vi "DC Basic Measure.vi"(4 "Channel 2":bool, 5 "Voltmeter 2 Address":string="8", 6 "Channel 1":bool=TRUE, 7 "Voltmeter 1 Address":string="7", 9 "Period (s)":string="1", 10 "Amplitude (A)":string="1e-8") -> (0 "STD 2":dbl=0.00015789614384998, 1 "Resistance 2":dbl=0.023133111600000002, 2 "STD 1":dbl=1.1063759259570055e-05, 3 "Resistance 1":dbl=0.04676234421500001)   [LabVIEW 2020]
uses:
  <vilib>/Instr/_visa.llb/GPIB Status Boolean Array.ctl
panel:
  out "Buffer 2 Data":dbl[][](array[numeric])=[[0.0, 1.69853343e-06], [0.05, 2.29085744e-06], [0.101, 2.2689427e-06], [0.152, 2.25641999e-06], [0.203, 2.27896086e-06], [0.254, 2.27332565e-06], [0.305, 2.24828023e-06], [0.356, 2.26142908e-06], [0.407, 2.27708246e-06], [0.458, 2.26268135e-06], [0.509, 2.28146541e-06], [0.56, 2.27520405e-06], [0.611, 2.25266318e-06], [0.662, 2.27207338e-06], [0.713, 2.26268135e-06], [0.764, 2.26455975e-06], [0.815, 2.27457792e-06], [0.866, 2.25892453e-06], [0.917, 2.28021313e-06], [0.968, 2.27144724e-06], [1.019, 2.2495325e-06], [1.07, 2.24201888e-06], [1.121, 2.2476541e-06], [1.172, 2.23763593e-06], [1.223, 2.25203705e-06], [1.274, 2.22260869e-06], [1.325, 2.25892453e-06], [1.376, 2.2689427e-06], [1.427, 2.23262685e-06], [1.478, 1.17257976e-06], [1.529, -2.35755925e-06], [1.58, -2.36006378e-06], [1.631, -2.37696934e-06], [1.681, -2.35192407e-06], [1.731, -2.35630699e-06], [1.781, -2.34628888e-06], [1.832, -2.35881152e-06], [1.882, -2.33188785e-06], [1.932, -2.33814917e-06], [1.982, -2.34941954e-06], [2.032, -2.3368969e-06], [2.083, -2.3782216e-06], [2.133, -2.36131604e-06], [2.183, -2.33752304e-06], [2.233, -2.36256831e-06], [2.283, -2.38135226e-06], [2.333, -2.36757736e-06], [2.384, -2.36068991e-06], [2.434, -2.37133415e-06], [2.484, -2.3782216e-06], [2.534, -2.3763432e-06], [2.584, -2.37696934e-06], [2.635, -2.37133415e-06], [2.685, -2.40264074e-06], [2.735, -2.37321255e-06], [2.785, -2.3801e-06], [2.835, -2.37947386e-06], [2.885, -2.38636131e-06], [2.935, -2.36882962e-06], [2.985, -1.36075749e-06], [3.035, -5.33931926e-08], [3.085, -3.6487539e-08]]
  out "Buffer 2 Plot":cluster{dbl[], dbl[]}(graph)={[0.0, 0.05, 0.101, 0.152, 0.203, 0.254, 0.305, 0.356, 0.407, 0.458, 0.509, 0.56, 0.611, 0.662, 0.713, 0.764, 0.815, 0.866, 0.917, 0.968, 1.019, 1.07, 1.121, 1.172, 1.223, 1.274, 1.325, 1.376, 1.427, 1.478, 1.529, 1.58, 1.631, 1.681, 1.731, 1.781, 1.832, 1.882, 1.932, 1.982, 2.032, 2.083, 2.133, 2.183, 2.233, 2.283, 2.333, 2.384, 2.434, 2.484, 2.534, 2.584, 2.635, 2.685, 2.735, 2.785, 2.835, 2.885, 2.935, 2.985, 3.035, 3.085], [1.69853343e-06, 2.29085744e-06, 2.2689427e-06, 2.25641999e-06, 2.27896086e-06, 2.27332565e-06, 2.24828023e-06, 2.26142908e-06, 2.27708246e-06, 2.26268135e-06, 2.28146541e-06, 2.27520405e-06, 2.25266318e-06, 2.27207338e-06, 2.26268135e-06, 2.26455975e-06, 2.27457792e-06, 2.25892453e-06, 2.28021313e-06, 2.27144724e-06, 2.2495325e-06, 2.24201888e-06, 2.2476541e-06, 2.23763593e-06, 2.25203705e-06, 2.22260869e-06, 2.25892453e-06, 2.2689427e-06, 2.23262685e-06, 1.17257976e-06, -2.35755925e-06, -2.36006378e-06, -2.37696934e-06, -2.35192407e-06, -2.35630699e-06, -2.34628888e-06, -2.35881152e-06, -2.33188785e-06, -2.33814917e-06, -2.34941954e-06, -2.3368969e-06, -2.3782216e-06, -2.36131604e-06, -2.33752304e-06, -2.36256831e-06, -2.38135226e-06, -2.36757736e-06, -2.36068991e-06, -2.37133415e-06, -2.3782216e-06, -2.3763432e-06, -2.37696934e-06, -2.37133415e-06, -2.40264074e-06, -2.37321255e-06, -2.3801e-06, -2.37947386e-06, -2.38636131e-06, -2.36882962e-06, -1.36075749e-06, -5.33931926e-08, -3.6487539e-08]}
  out "Voltage 2":dbl[](array[numeric])=[2.31331116e-06, 1.5789614384998e-08]
  out "Python error 2":errorcluster
  out "T2":dbl[](array[numeric])=[0.0, 0.05, 0.101, 0.152, 0.203, 0.254, 0.305, 0.356, 0.407, 0.458, 0.509, 0.56, 0.611, 0.662, 0.713, 0.764, 0.815, 0.866, 0.917, 0.968, 1.019, 1.07, 1.121, 1.172, 1.223, 1.274, 1.325, 1.376, 1.427, 1.478, 1.529, 1.58, 1.631, 1.681, 1.731, 1.781, 1.832, 1.882, 1.932, 1.982, 2.032, 2.083, 2.133, 2.183, 2.233, 2.283, 2.333, 2.384, 2.434, 2.484, 2.534, 2.584, 2.635, 2.685, 2.735, 2.785, 2.835, 2.885, 2.935, 2.985, 3.035, 3.085]
  out "V2":dbl[](array[numeric])=[1.69853343e-06, 2.29085744e-06, 2.2689427e-06, 2.25641999e-06, 2.27896086e-06, 2.27332565e-06, 2.24828023e-06, 2.26142908e-06, 2.27708246e-06, 2.26268135e-06, 2.28146541e-06, 2.27520405e-06, 2.25266318e-06, 2.27207338e-06, 2.26268135e-06, 2.26455975e-06, 2.27457792e-06, 2.25892453e-06, 2.28021313e-06, 2.27144724e-06, 2.2495325e-06, 2.24201888e-06, 2.2476541e-06, 2.23763593e-06, 2.25203705e-06, 2.22260869e-06, 2.25892453e-06, 2.2689427e-06, 2.23262685e-06, 1.17257976e-06, -2.35755925e-06, -2.36006378e-06, -2.37696934e-06, -2.35192407e-06, -2.35630699e-06, -2.34628888e-06, -2.35881152e-06, -2.33188785e-06, -2.33814917e-06, -2.34941954e-06, -2.3368969e-06, -2.3782216e-06, -2.36131604e-06, -2.33752304e-06, -2.36256831e-06, -2.38135226e-06, -2.36757736e-06, -2.36068991e-06, -2.37133415e-06, -2.3782216e-06, -2.3763432e-06, -2.37696934e-06, -2.37133415e-06, -2.40264074e-06, -2.37321255e-06, -2.3801e-06, -2.37947386e-06, -2.38636131e-06, -2.36882962e-06, -1.36075749e-06, -5.33931926e-08, -3.6487539e-08]
  out "Write Status 2":T1=[FALSE, FALSE, FALSE, FALSE, FALSE, FALSE, FALSE, FALSE, TRUE, FALSE, FALSE, FALSE, FALSE, FALSE, FALSE, FALSE]
  out "error out 2":errorcluster
  out "Read Status 2":T1=[FALSE, FALSE, FALSE, FALSE, FALSE, FALSE, FALSE, FALSE, TRUE, FALSE, FALSE, FALSE, FALSE, TRUE, FALSE, FALSE]
  out "Buffer 1 Data":dbl[][](array[numeric])=[[0.0, 9.9e+37], [0.014, 9.9e+37], [0.026, 9.9e+37], [0.04, 9.9e+37], [0.052, 9.9e+37], [0.067, 9.9e+37], [0.079, 9.9e+37], [0.093, 9.9e+37], [0.105, 9.9e+37], [0.12, 9.9e+37], [0.132, 9.9e+37], [0.146, 9.9e+37], [0.158, 9.9e+37], [0.172, 9.9e+37], [0.184, 9.9e+37], [0.199, 9.9e+37], [0.211, 9.9e+37], [0.225, 9.9e+37], [0.237, 9.9e+37], [0.251, 9.9e+37], [0.263, 9.9e+37], [0.277, 9.9e+37], [0.289, 9.9e+37], [0.304, 9.9e+37], [0.316, 9.9e+37], [0.33, 9.9e+37], [0.342, 9.9e+37], [0.356, 9.9e+37], [0.368, 9.9e+37], [0.383, 9.9e+37], [0.395, 9.9e+37], [0.409, 9.9e+37], [0.422, 9.9e+37], [0.437, 9.9e+37], [0.449, 9.9e+37], [0.463, 9.9e+37], [0.475, 9.9e+37], [0.49, 9.9e+37], [0.502, 9.9e+37], [0.516, 9.9e+37], [0.528, 9.9e+37], [0.542, 9.9e+37], [0.554, 9.9e+37], [0.568, 9.9e+37], [0.58, 9.9e+37], [0.595, 9.9e+37], [0.607, 9.9e+37], [0.621, 9.9e+37], [0.633, 9.9e+37], [0.647, 9.9e+37], [0.659, 9.9e+37], [0.674, 9.9e+37], [0.686, 9.9e+37], [0.7, 9.9e+37], [0.712, 9.9e+37], [0.726, 9.9e+37], [0.738, 9.9e+37], [0.753, 9.9e+37], [0.765, 9.9e+37], [0.779, 9.9e+37], [0.791, 9.9e+37], [0.805, 9.9e+37]]
  out "Buffer 1 Plot":cluster{dbl[], dbl[]}(graph)={[0.0, 0.014, 0.026, 0.04, 0.052, 0.067, 0.079, 0.093, 0.105, 0.12, 0.132, 0.146, 0.158, 0.172, 0.184, 0.199, 0.211, 0.225, 0.237, 0.251, 0.263, 0.277, 0.289, 0.304, 0.316, 0.33, 0.342, 0.356, 0.368, 0.383, 0.395, 0.409, 0.422, 0.437, 0.449, 0.463, 0.475, 0.49, 0.502, 0.516, 0.528, 0.542, 0.554, 0.568, 0.58, 0.595, 0.607, 0.621, 0.633, 0.647, 0.659, 0.674, 0.686, 0.7, 0.712, 0.726, 0.738, 0.753, 0.765, 0.779, 0.791, 0.805], [9.9e+37, 9.9e+37, 9.9e+37, 9.9e+37, 9.9e+37, 9.9e+37, 9.9e+37, 9.9e+37, 9.9e+37, 9.9e+37, 9.9e+37, 9.9e+37, 9.9e+37, 9.9e+37, 9.9e+37, 9.9e+37, 9.9e+37, 9.9e+37, 9.9e+37, 9.9e+37, 9.9e+37, 9.9e+37, 9.9e+37, 9.9e+37, 9.9e+37, 9.9e+37, 9.9e+37, 9.9e+37, 9.9e+37, 9.9e+37, 9.9e+37, 9.9e+37, 9.9e+37, 9.9e+37, 9.9e+37, 9.9e+37, 9.9e+37, 9.9e+37, 9.9e+37, 9.9e+37, 9.9e+37, 9.9e+37, 9.9e+37, 9.9e+37, 9.9e+37, 9.9e+37, 9.9e+37, 9.9e+37, 9.9e+37, 9.9e+37, 9.9e+37, 9.9e+37, 9.9e+37, 9.9e+37, 9.9e+37, 9.9e+37, 9.9e+37, 9.9e+37, 9.9e+37, 9.9e+37, 9.9e+37, 9.9e+37]}
  in  "Python Support File":path=path "C:/Users/QDUser/Desktop/LabVIEW Programs/PPMS Interface/lib/PPMS External Control Support.py"
  out "Voltage 1":dbl[](array[numeric])=[0.0, 0.014, 0.026, 0.04, 0.052, 0.067, 0.079, 0.093, 0.105, 0.12, 0.132, 0.146, 0.158, 0.172, 0.184, 0.199, 0.211, 0.225, 0.237, 0.251, 0.263, 0.277, 0.289, 0.304, 0.316, 0.33, 0.342, 0.356, 0.368, 0.383, 0.395, 0.409, 0.422, 0.437, 0.449, 0.463, 0.475, 0.49, 0.502, 0.516, 0.528, 0.542, 0.554, 0.568, 0.58, 0.595, 0.607, 0.621, 0.633, 0.647, 0.659, 0.674, 0.686, 0.7, 0.712, 0.726, 0.738, 0.753, 0.765, 0.779, 0.791, 0.805]
  out "Python error":errorcluster={"status"=TRUE, "code"=1671, "source"="Python Node in DC Transport Measure.vi<APPEND>\n\nModule Path: C:\\Users\\qmgmit\\Desktop\\Shivam\\PPMS External Control\\lib\\PPMS External Control Support.pyc\nFunction Name: process_DC_buffer\nPython returned the following error: <type 'exceptions.IndexError'>\nindex 62 is out of bounds for axis 0 with size 62\n\n\nCall Stack information:\n  File \"C:\\Users\\qmgmit\\Desktop\\Shivam\\PPMS External Control\\lib\\PPMS External Control Support.py\", line 22, in process_DC_buffer\n    if (time[index]>tpos_min):\n\nIndexError: index 62 is out of bounds for axis 0 with size 62\n"}
  out "T1":dbl[](array[numeric])=[0.0, 0.014, 0.026, 0.04, 0.052, 0.067, 0.079, 0.093, 0.105, 0.12, 0.132, 0.146, 0.158, 0.172, 0.184, 0.199, 0.211, 0.225, 0.237, 0.251, 0.263, 0.277, 0.289, 0.304, 0.316, 0.33, 0.342, 0.356, 0.368, 0.383, 0.395, 0.409, 0.422, 0.437, 0.449, 0.463, 0.475, 0.49, 0.502, 0.516, 0.528, 0.542, 0.554, 0.568, 0.58, 0.595, 0.607, 0.621, 0.633, 0.647, 0.659, 0.674, 0.686, 0.7, 0.712, 0.726, 0.738, 0.753, 0.765, 0.779, 0.791, 0.805]
  out "V1":dbl[](array[numeric])=[9.9e+37, 9.9e+37, 9.9e+37, 9.9e+37, 9.9e+37, 9.9e+37, 9.9e+37, 9.9e+37, 9.9e+37, 9.9e+37, 9.9e+37, 9.9e+37, 9.9e+37, 9.9e+37, 9.9e+37, 9.9e+37, 9.9e+37, 9.9e+37, 9.9e+37, 9.9e+37, 9.9e+37, 9.9e+37, 9.9e+37, 9.9e+37, 9.9e+37, 9.9e+37, 9.9e+37, 9.9e+37, 9.9e+37, 9.9e+37, 9.9e+37, 9.9e+37, 9.9e+37, 9.9e+37, 9.9e+37, 9.9e+37, 9.9e+37, 9.9e+37, 9.9e+37, 9.9e+37, 9.9e+37, 9.9e+37, 9.9e+37, 9.9e+37, 9.9e+37, 9.9e+37, 9.9e+37, 9.9e+37, 9.9e+37, 9.9e+37, 9.9e+37, 9.9e+37, 9.9e+37, 9.9e+37, 9.9e+37, 9.9e+37, 9.9e+37, 9.9e+37, 9.9e+37, 9.9e+37, 9.9e+37, 9.9e+37]
  out "Write Status":T1=[FALSE, FALSE, FALSE, FALSE, FALSE, FALSE, FALSE, FALSE, TRUE, FALSE, FALSE, FALSE, FALSE, FALSE, FALSE, FALSE]
  in  "Byte Count":i32=2000
  out "error out":errorcluster
  out "Read Status":T1=[FALSE, FALSE, FALSE, FALSE, FALSE, FALSE, FALSE, FALSE, TRUE, FALSE, FALSE, FALSE, FALSE, TRUE, FALSE, FALSE]
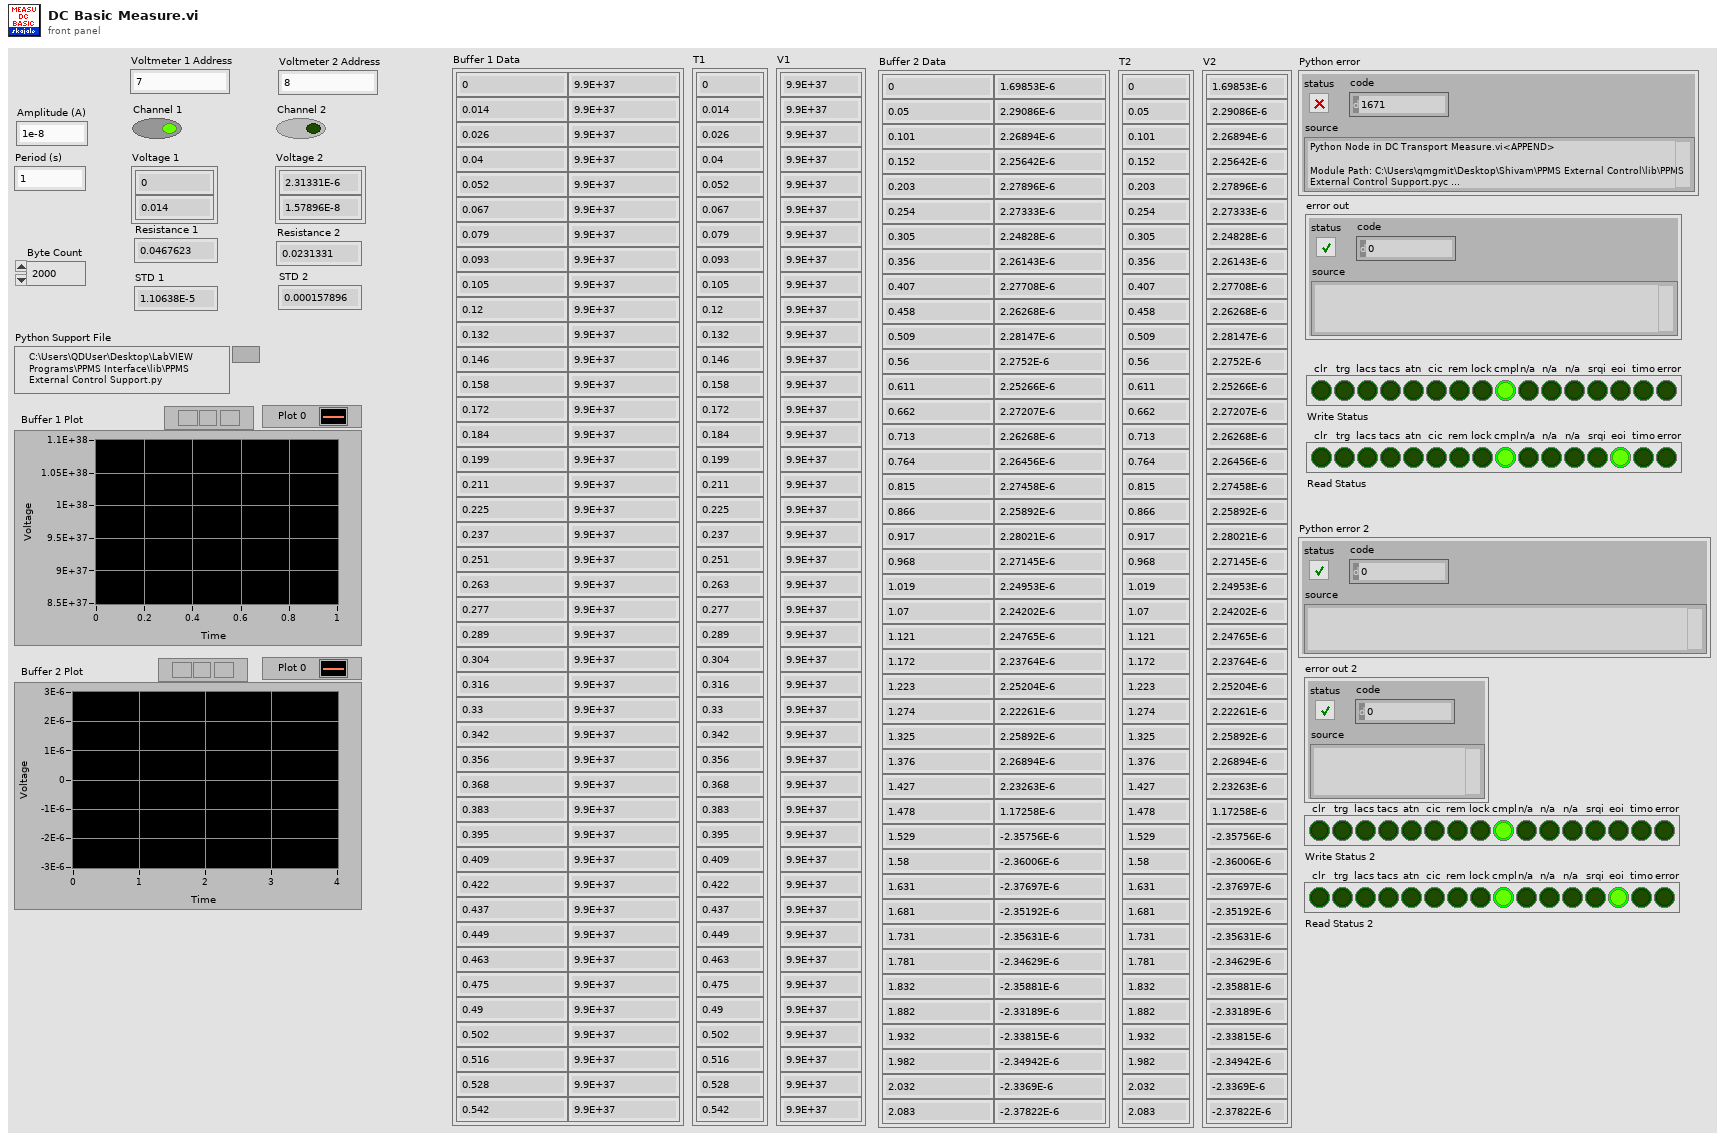
[diagram p1: front panel]
types:
  T1 = typedef "GPIB Status Boolean Array.ctl" = bool[]
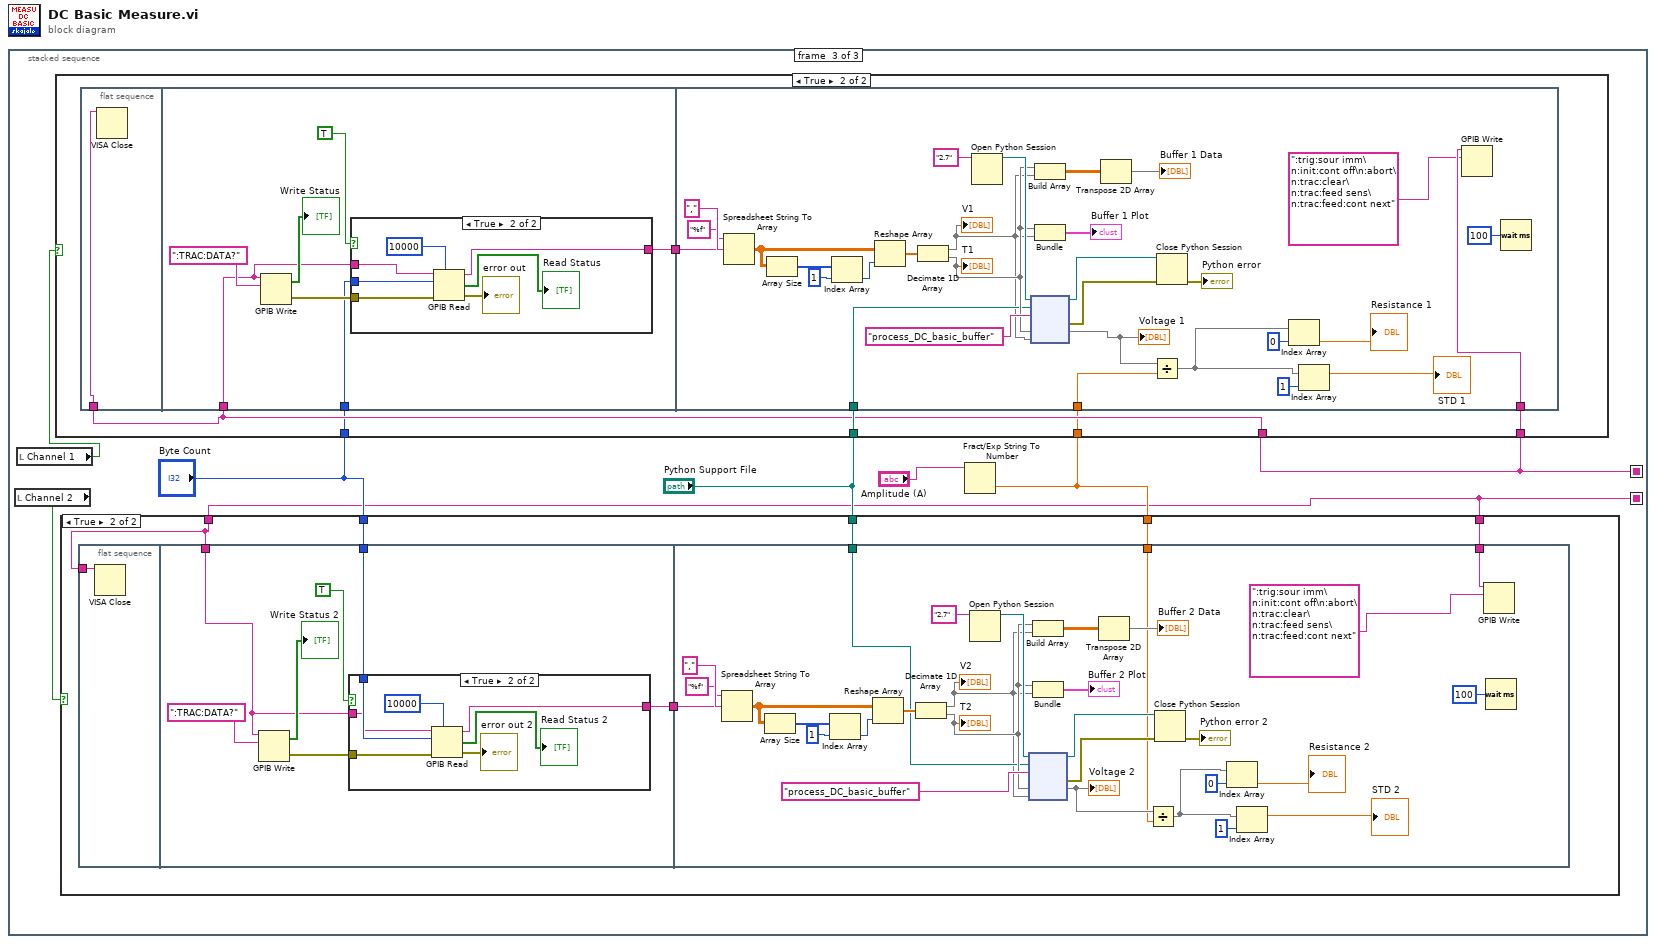
[diagram p0: block diagram]
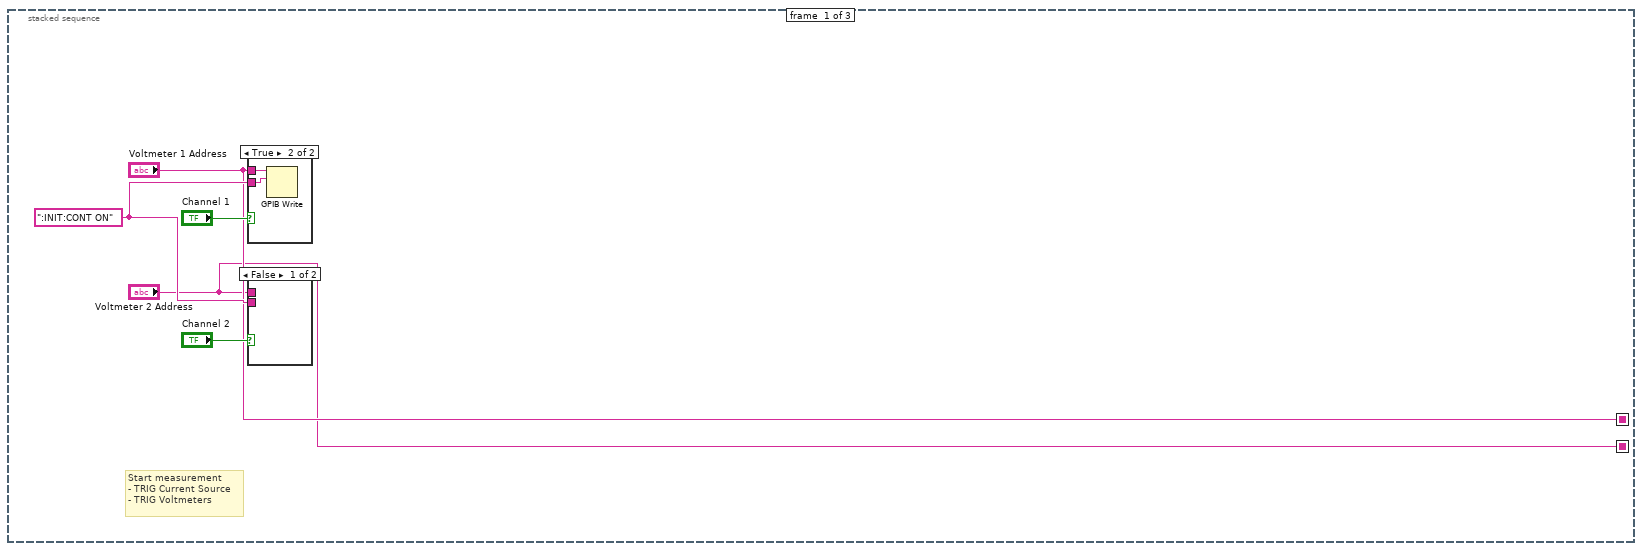
[diagram p2: hidden frame]
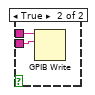
[diagram p4: hidden frame]
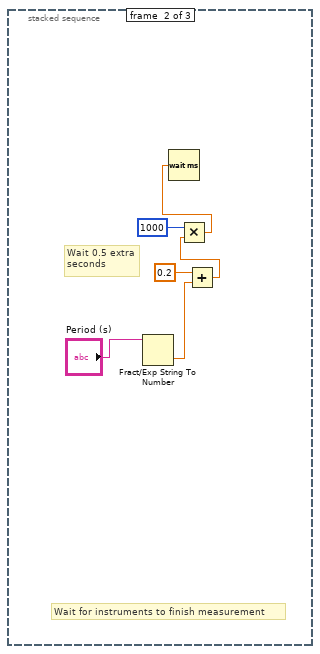
[diagram p5: hidden frame]
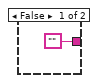
[diagram p7: hidden frame]
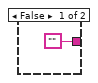
[diagram p9: hidden frame]
diagram:
  n1 = stacked-sequence {
    seq-local: ["Voltmeter 1 Address" _ _] -> [_ _ w17]
    seq-local: ["Voltmeter 2 Address" _ _] -> [_ _ w16]
    frame #0 {
      w3 = ":INIT:CONT ON" ("data")
      # "Start measurement\n- TRIG Current Source\n- TRIG Voltmeters"
      n2 = case shown="True" "Channel 1" {
        tunnel: "Voltmeter 1 Address" -> [_ w7]
        tunnel: w3 -> [_ w6]
        frame False {
        }
        frame True {
          n3 = GPIB Write(0:w7, 1:w6) -> ()  [unwired: 3 in, 2 out]
        }
      }
      n4 = case shown="False" "Channel 2" {
        tunnel: "Voltmeter 2 Address" -> [_ w9]
        tunnel: w3 -> [_ w8]
        frame False {
        }
        frame True {
          n5 = GPIB Write(0:w9, 1:w8) -> ()  [unwired: 3 in, 2 out]
        }
      }
    }
    frame #1 {
      # "Wait for instruments to finish measurement"
      # "Wait 0.5 extra\nseconds"
      n6 = Fract/Exp String To Number(string="Period (s)") -> (number=w10:dbl)  [unwired: 3 in, 1 out]
      n7 = Add(x=0.2, y=w10) -> (x+y=w14:dbl)
      n8 = Multiply(x=1000, y=w14) -> (x*y=w12:dbl)
      n9 = Wait (ms)(milliseconds to wait=w12) -> ()  [unwired: 1 out]
    }
    frame #2 {
      n10 = local read "Channel 2"() -> (w22:bool)
      n11 = local read "Channel 1"() -> (w21:bool)
      n12 = Fract/Exp String To Number(string="Amplitude (A)") -> (number=w18:dbl)  [unwired: 3 in, 1 out]
      n13 = case shown="True" w21 {
        tunnel: "Python Support File" -> [_ w80]
        tunnel: w17 -> [_ w79]
        tunnel: "Byte Count" -> [_ w78]
        tunnel: w18 -> [_ w77]
        tunnel: w17 -> [_ w76]
        frame False {
        }
        frame True {
          n14 = flat-sequence {
            tunnel: w79 -> [w82]
            tunnel: [w85] -> w81
            tunnel: w79 -> [w83]
            tunnel: w78 -> [w84]
            tunnel: w81 -> [w110]
            tunnel: w80 -> [w109]
            tunnel: w77 -> [w107]
            tunnel: w76 -> [w101]
            frame #0 {
              n15 = VISA Close(VISA resource name=w82) -> ()  [unwired: 1 in, 1 out]
            }
            frame #1 {
              n16 = GPIB Write(0:w83, 1:":TRAC:DATA?" ("data")) -> (5:→"Write Status":bool[], 6:w88:errorcluster)  [unwired: 3 in]
              n17 = case shown="True" TRUE ("Query?") {
                tunnel: w88 -> [_ w96]
                tunnel: w84 -> [_ w93]
                tunnel: ["" w92] -> w85
                tunnel: w83 -> [_ w91]
                frame False {
                }
                frame True {
                  n18 = GPIB Read(0:w91, 1:w93, 3:w96, 4:10000 ("timeout ms (488.2 global)")) -> (5:w92:string, 6:→"Read Status":bool[], 7:→"error out":errorcluster)  [unwired: 1 in]
                }
              }
            }
            frame #2 {
              n19 = Spreadsheet String To Array(delimiter (Tab)=",", format string="%f", spreadsheet string=w110) -> (array=w126:dbl[][])  [unwired: 1 in]
              n20 = Array Size(array=w126) -> (size(s)=w125:i32[])
              n21 = Index Array(array=w125, index=1) -> (element=w123:i32)
              n22 = Reshape Array(w126, w123) -> (w122:dbl[])
              n23 = Decimate 1D Array(w122) -> (w98:dbl[], w113:dbl[])
              "T1" <- w113
              "V1" <- w98
              n24 = Open Python Session(python version="2.7" ("Python version")) -> (session out=w117:refnum<k35>)  [unwired: 2 in, 1 out]
              n25 = node(w117, w109, "process_DC_basic_buffer" ("Buffer Process Function"), w113, w98) -> (w115:refnum<k35>, w112:errorcluster, w108:dbl[])  [unwired: 2 in, 2 out]
              "Voltage 1" <- w108
              n26 = Build Array(w113, w98) -> (w121:dbl[][])
              n27 = Bundle(w113, w98) -> (→"Buffer 1 Plot":cluster{dbl[], dbl[]})  [unwired: 1 in]
              n28 = Transpose 2D Array(2D array=w121) -> (transposed array=→"Buffer 1 Data":dbl[][])
              n29 = Divide(x=w108, y=w107) -> (x/y=w104:dbl[])
              n30 = Close Python Session(session in=w115, error in=w112) -> (11:→"Python error":errorcluster)
              n31 = Index Array(array=w104, index=0) -> (element=→"Resistance 1":dbl)
              n32 = Index Array(array=w104, index=1) -> (element=→"STD 1":dbl)
              n33 = GPIB Write(0:w101, 1:":trig:sour imm\n:init:cont off\n:abort\n:trac:clear\n:trac:feed sens\n:trac:feed:cont next" ("data")) -> ()  [unwired: 3 in, 2 out]
              n34 = Wait (ms)(milliseconds to wait=u32 100) -> ()  [unwired: 1 out]
            }
          }
        }
      }
      n35 = case shown="True" w22 {
        tunnel: "Python Support File" -> [_ w28]
        tunnel: w16 -> [_ w27]
        tunnel: "Byte Count" -> [_ w26]
        tunnel: w18 -> [_ w25]
        tunnel: w16 -> [_ w24]
        frame False {
        }
        frame True {
          n36 = flat-sequence {
            tunnel: w27 -> [w30]
            tunnel: [w33] -> w29
            tunnel: w27 -> [w31]
            tunnel: w26 -> [w32]
            tunnel: w29 -> [w58]
            tunnel: w28 -> [w57]
            tunnel: w25 -> [w55]
            tunnel: w24 -> [w49]
            frame #0 {
              n37 = VISA Close(VISA resource name=w30) -> ()  [unwired: 1 in, 1 out]
            }
            frame #1 {
              n38 = GPIB Write(0:w31, 1:":TRAC:DATA?" ("data")) -> (5:→"Write Status 2":bool[], 6:w36:errorcluster)  [unwired: 3 in]
              n39 = case shown="True" TRUE ("Query?") {
                tunnel: w36 -> [_ w44]
                tunnel: ["" w41] -> w33
                tunnel: w32 -> [_ w40]
                tunnel: w31 -> [_ w39]
                frame False {
                }
                frame True {
                  n40 = GPIB Read(0:w39, 1:w40, 3:w44, 4:10000 ("timeout ms (488.2 global)")) -> (5:w41:string, 6:→"Read Status 2":bool[], 7:→"error out 2":errorcluster)  [unwired: 1 in]
                }
              }
            }
            frame #2 {
              n41 = Spreadsheet String To Array(delimiter (Tab)=",", format string="%f", spreadsheet string=w58) -> (array=w74:dbl[][])  [unwired: 1 in]
              n42 = Array Size(array=w74) -> (size(s)=w73:i32[])
              n43 = Index Array(array=w73, index=1) -> (element=w71:i32)
              n44 = Reshape Array(w74, w71) -> (w70:dbl[])
              n45 = Decimate 1D Array(w70) -> (w46:dbl[], w61:dbl[])
              "T2" <- w61
              "V2" <- w46
              n46 = Open Python Session(python version="2.7" ("Python version")) -> (session out=w65:refnum<k35>)  [unwired: 2 in, 1 out]
              n47 = node(w65, w57, "process_DC_basic_buffer" ("Buffer Process Function"), w61, w46) -> (w63:refnum<k35>, w60:errorcluster, w56:dbl[])  [unwired: 2 in, 2 out]
              "Voltage 2" <- w56
              n48 = Build Array(w61, w46) -> (w69:dbl[][])
              n49 = Bundle(w61, w46) -> (→"Buffer 2 Plot":cluster{dbl[], dbl[]})  [unwired: 1 in]
              n50 = Transpose 2D Array(2D array=w69) -> (transposed array=→"Buffer 2 Data":dbl[][])
              n51 = Divide(x=w56, y=w55) -> (x/y=w50:dbl[])
              n52 = Close Python Session(session in=w63, error in=w60) -> (11:→"Python error 2":errorcluster)
              n53 = Index Array(array=w50, index=0) -> (element=→"Resistance 2":dbl)
              n54 = Index Array(array=w50, index=1) -> (element=→"STD 2":dbl)
              n55 = GPIB Write(0:w49, 1:":trig:sour imm\n:init:cont off\n:abort\n:trac:clear\n:trac:feed sens\n:trac:feed:cont next" ("data")) -> ()  [unwired: 3 in, 2 out]
              n56 = Wait (ms)(milliseconds to wait=u32 100) -> ()  [unwired: 1 out]
            }
          }
        }
      }
    }
  }
